vi "Host Main.vi"() -> ()   [LabVIEW 2015]
doc: "This application launches and executes the Tag Bus Data framework configuration for the specified target alias. This is a simple example of the framework API functions, but may also be a suitable starting point for a Host UI or Thick Client that is running a local version of the framework."
uses:
  <vilib>/NI/Module Execution Interface/Engine Runtime/Execution States.ctl
  <vilib>/NI/Module Execution Interface/Engine Runtime/Fault.ctl
  <vilib>/NI/Tag Bus Module Framework/runtime/error classification.ctl
  <vilib>/NI/Module Execution Interface/Engine Runtime/Engine Runtime Interface.lvclass
  <vilib>/NI/DCAF/Tag Editor Core/Framework Configuration Classes/target runtime/PL_Target Runtime.lvclass
  <vilib>/NI/Tag Bus Module Framework/FPGA manager/FPGA manager.lvlib
  <vilib>/rvi/interface/nirviOpenFPGA/nirviOpenFPGA.xnode
  <vilib>/userdefined/High Color/nirio_resource_hc.ctl
  <vilib>/NI/Tag Bus Module Framework/FPGA manager/methods.ctl
  <vilib>/NI/Tag Bus Module Framework/runtime/TBM module execution interface.lvclass
panel:
  in  "configuration file path":path=path "C:/Users/blueuser/Desktop/Hands On/Hands-On_1/myExercises/Temperature Controller/SimulatedSystem.pcfg"
  in  "target alias":string="PC"
  out "engine status":T4(array[cluster])
  in  "stop":bool
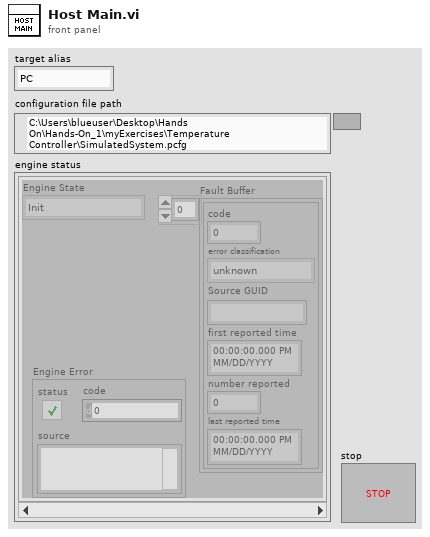
[diagram p1: front panel]
types:
  T1 = typedef "Engine Runtime Interface.lvclass/Execution States.ctl" = enum16{"Init", "Pre-Operational", "Safe-Operational", "Operational", "Stopped"}
  T2 = typedef "Engine Runtime Interface.lvclass/Fault.ctl" = cluster{"code":i32, "error classification":T3, "Source GUID":string, "first reported time":timestamp, "number reported":u32, "last reported time":timestamp}
  T3 = typedef "TBM module execution interface.lvclass/error classification.ctl" = enum16{"unknown", "none", "trivial", "recoverable", "critical"}
  T4 = cluster{"Engine State":T1, "Fault Buffer":T2[], "Engine Error":errorcluster}[]
  T5 = typedef "FPGA manager.lvlib/methods.ctl" = enum16{"initialize bitfile", "cache bitfile", "locate bitfile", "close bitfile", "clear manager"}
  T6 = typedef "nirio_resource_hc.ctl" = tag
  T7 = cluster{"Engine State":T1, "Fault Buffer":T2[], "Engine Error":errorcluster}
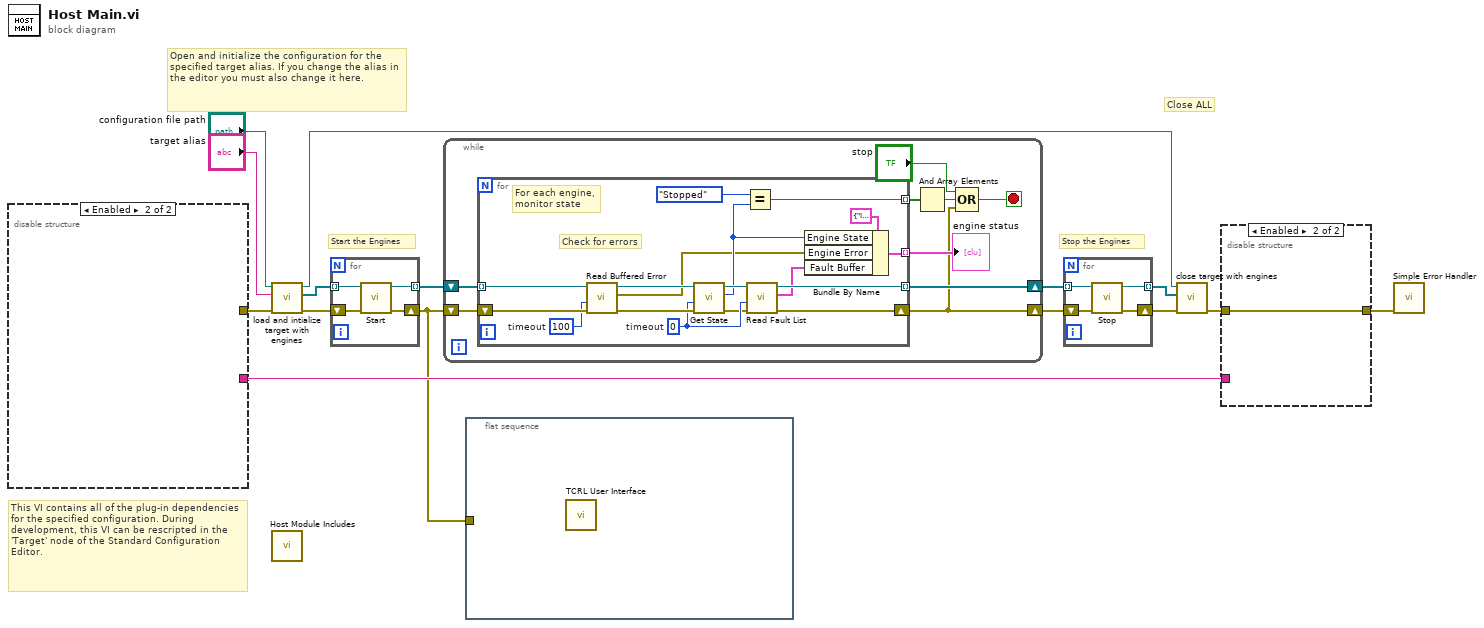
[diagram p0: block diagram]
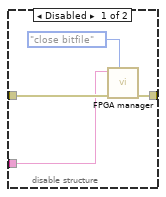
[diagram p2: hidden frame]
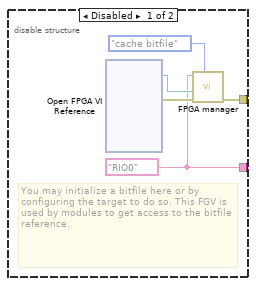
[diagram p3: hidden frame]
diagram:
  # "Start the Engines"
  # "Open and initialize the configuration for the specified target alias. If you change the alias in the editor you must also change it here."
  # "Close ALL"
  # "Stop the Engines"
  # "This VI contains all of the plug-in dependencies for the specified configuration. During development, this VI can be rescripted in the 'Target' node of the Standard Configuration Editor."
  n1 = disable-structure shown="Enabled" {
    disable-tunnel: [w20 _] -> w5
    disable-tunnel: [w16 _] -> w4
    frame Disabled {
      w16 = T6 "RIO0" ("RIO resource")
      # "You may initialize a bitfile here or by configuring the target to do so. This FGV is used by modules to get access to the bitfile reference."
      n2 = xnode "Open FPGA VI Reference"() -> ("FPGA VI Reference Out"=w18:refnum<k20>, "error out"=w19:errorcluster)  [unwired: 2 in]
      n3 = call <vilib>:"FPGA manager.vi"("action"=methods."cache bitfile", "error in"=w19, "bitfile to cache"=w18, "RIO resource"=w16) -> ("error out"=w20:errorcluster)  [unwired: 5 in, 2 out]
    }
    frame Enabled {
    }
  }
  n4 = call <vilib>:"load and intialize target with engines.vi"("error in"=w5, "target alias"="target alias", "file path"="configuration file path") -> ("error out"=w12:errorcluster, "engine runtime interfaces"=w11:refnum<class "Engine Runtime Interface.lvclass">[], "target runtime"=w8:refnum<class "PL_Target Runtime.lvclass">)  [unwired: 6 in]
  n5 = call "Host Module Includes.vi"() -> ()  [unwired: 12 in]
  n6 = for {
    tunnel: [w24] -> w15 mode=indexing
    tunnel: w11 -> [w21] mode=indexing
    shift-right: [w23] -> w2
    shift-left: w12 -> [w22]
    n7 = call-dynamic "Start.vi"("error in"=w22, "Engine Runtime Interface in"=w21) -> ("error out"=w23:errorcluster, "Engine Runtime Interface out"=w24:refnum<class "Engine Runtime Interface.lvclass">)  [unwired: 8 in]
  }
  n8 = while {
    shift-right: [w31] -> w14
    shift-left: w15 -> [w33]
    shift-right: [w25] -> w13
    shift-left: w2 -> [w32]
    stop <- w29 stop-if-true
    n9 = for {
      tunnel: w33 -> [w50] mode=indexing
      tunnel: [w42] -> w31 mode=indexing
      tunnel: [w45] -> w27 mode=indexing
      shift-right: [w41] -> w25
      shift-left: w32 -> [w49]
      tunnel: [w37] -> w28 mode=indexing
      w40 = 0  # timeout
      w44 = 100  # timeout
      # "For each engine, \nmonitor state"
      # "Check for errors"
      n10 = call-dynamic "Read Buffered Error.vi"("error in"=w49, "timeout in ms (0)"=w44, "Engine Runtime Interface in"=w50) -> ("error out"=w47:errorcluster, "Engine Error"=w35:errorcluster, "Engine Runtime Interface out"=w48:refnum<class "Engine Runtime Interface.lvclass">)  [unwired: 6 in]
      n11 = call-dynamic "Get State.vi"("error in"=w47, "timeout (-1)"=w40, "Engine Runtime Interface in"=w48) -> ("error out"=w34:errorcluster, "Engine State"=w39:T1, "Engine Runtime Interface out"=w43:refnum<class "Engine Runtime Interface.lvclass">)  [unwired: 6 in]
      n12 = Equal?(x=Execution_States."Stopped" ("Engine State"), y=w39) -> (x = y?=w45:bool)
      n13 = call-dynamic "Read Fault List.vi"("error in"=w34, "timeout (-1)"=w40, "Engine Runtime Interface in"=w43) -> ("error out"=w41:errorcluster, "faults"=w38:T2[], "Engine Runtime Interface out"=w42:refnum<class "Engine Runtime Interface.lvclass">)  [unwired: 6 in]
      n14 = Bundle By Name(cluster=T7 {"Engine State"=enum."Init", "Fault Buffer"=[], "Engine Error"={"status"=FALSE, "code"=0, "source"=""}}, "Engine State"=w39, "Engine Error"=w35, "Fault Buffer"=w38) -> (w37:T7)
    }
    "engine status" <- w28
    n15 = And Array Elements(Boolean array=w27) -> (logical AND=w26:bool)
    n16 = Compound Arithmetic op=OR("stop", w26, w25) -> (w29:bool)
  }
  n17 = flat-sequence {
    tunnel: w2 -> [_]
    frame #0 {
      n18 = call "TCRL User Interface.vi"() -> ()  [unwired: 12 in]
    }
  }
  n19 = for {
    tunnel: w14 -> [w54] mode=indexing
    shift-right: [w51] -> w7
    shift-left: w13 -> [w53]
    tunnel: [w52] -> w9 mode=indexing
    n20 = call-dynamic "Stop.vi"("error in"=w53, "Engine Runtime Interface in"=w54) -> ("error out"=w51:errorcluster, "Engine Runtime Interface out"=w52:refnum<class "Engine Runtime Interface.lvclass">)  [unwired: 8 in]
  }
  n21 = call <vilib>:"close target with engines.vi"("error in"=w7, "Engine Runtime Interfaces"=w9, "Target Runtime"=w8) -> ("error out"=w3:errorcluster)  [unwired: 8 in]
  n22 = disable-structure shown="Enabled" {
    disable-tunnel: [w57 w59] -> w1
    disable-tunnel: w3 -> [w58 w59]
    disable-tunnel: w4 -> [w55 _]
    frame Disabled {
      n23 = call <vilib>:"FPGA manager.vi"("action"=methods."close bitfile", "error in"=w58, "RIO resource"=w55) -> ("error out"=w57:errorcluster)  [unwired: 6 in, 2 out]
    }
    frame Enabled {
    }
  }
  n24 = call <vilib>:"Simple Error Handler.vi"("error in (no error)"=w1) -> ()  [unwired: 4 in, 5 out]
